vi "dev_arraytesting.vi"() -> ()   [LabVIEW 2020]
panel:
  in  "Search Timestamp":u32
  out "sum":dbl
  out "subarray":dbl[](array[numeric])
  out "min index(es)":i32
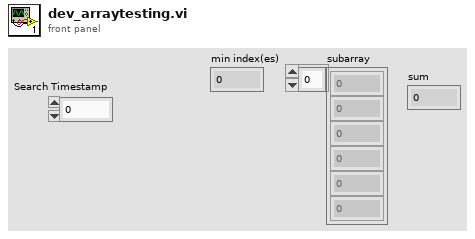
[diagram p1: front panel]
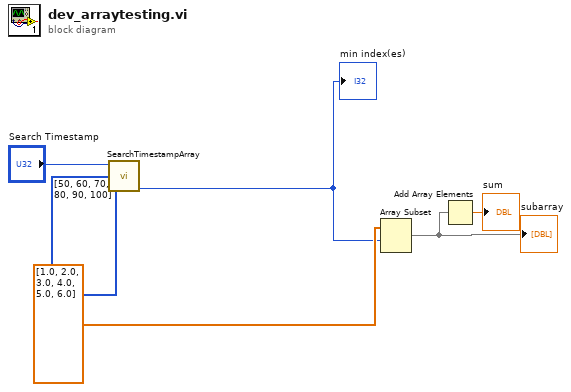
[diagram p0: block diagram]
diagram:
  n1 = call "SearchTimestampArray.vi"("Timestamp Array"=u32[] [50, 60, 70, 80, 90, 100], "Search Timestamp"="Search Timestamp") -> ("Index of Minimum"=w3:i32)  [unwired: 8 in, 1 out]
  "min index(es)" <- w3
  n2 = Array Subset(array=dbl[] [1.0, 2.0, 3.0, 4.0, 5.0, 6.0], index=w3) -> (w5:dbl[])  [unwired: 1 in]
  "subarray" <- w5
  n3 = Add Array Elements(numeric array=w5) -> (sum=→"sum":dbl)
